vi "TDMS.vi"(10 "Guardar en:":path, 11 "Array":dbl[][](array[numeric])) -> ()   [LabVIEW 2017]
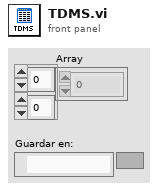
[diagram p1: front panel]
types:
  T1 = enum16{"open", "open or create", "create or replace", "create", "open (read-only)"}
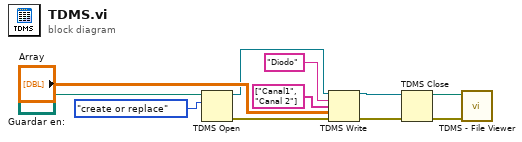
[diagram p0: block diagram]
diagram:
  n1 = TDMS Open(10:T1."create or replace" ("operation (0:open)"), 11:"Guardar en:") -> (0:w4:errorcluster, 3:w7:refnum<k34>)  [unwired: 5 in]
  n2 = TDMS Write(0:w7, 5:"Diodo" ("group name in (Untitled)"), 7:string[] ["Canal1", "Canal 2"] ("channel name(s) in (Untitled)"), 9:"Array", 11:w4) -> (4:w6:refnum<k34>, 15:w5:errorcluster)  [unwired: 1 in, 2 out]
  n3 = TDMS Close(8:w5, 11:w6) -> (0:w9:errorcluster, 3:w10:path)
  n4 = call <vilib>:"TDMS - File Viewer.vi"("error in (no error)"=w9, "file path"=w10) -> ()  [unwired: 4 in, 2 out]
